vi "DO.Write.vi"(8 "error in (no error)":errorcluster, 11 "DO Data":cluster{"DO Name":string, "DO Value":variant}[](array[cluster])) -> (0 "error out":errorcluster)   [LabVIEW 2019]
doc: "Writes an array of Digital Outputs to hardware, where \"DO Name\" is the name of the channel and \"DO Value\" is the value to write."
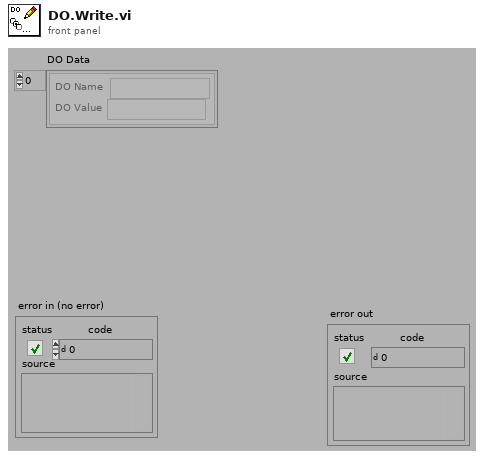
[diagram p1: front panel]
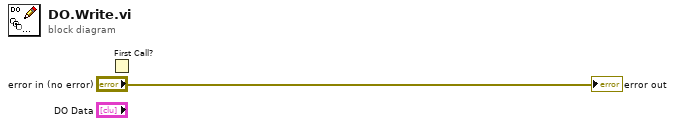
[diagram p0: block diagram]
diagram:
  n1 = First Call?() -> ()  [unwired: 1 out]
  "error out" <- "error in (no error)"
